vi "Profile Auton - Shooting Mode.vi"(8 "error in (no error)":errorcluster, 10 "Time (s)":dbl, 11 "Shooting Mode":T1(ring)) -> (0 "error out":errorcluster)   [LabVIEW 2017]
uses:
  <vilib>/Rock Robotics/WPI/Solenoid/WPI_SolenoidValue.ctl
  <vilib>/Rock Robotics/WPI/Utilities/WPI_GetSetVariantRefNum.vi
  <vilib>/Rock Robotics/WPI/Solenoid/WPI_SolenoidSetEnum.vi
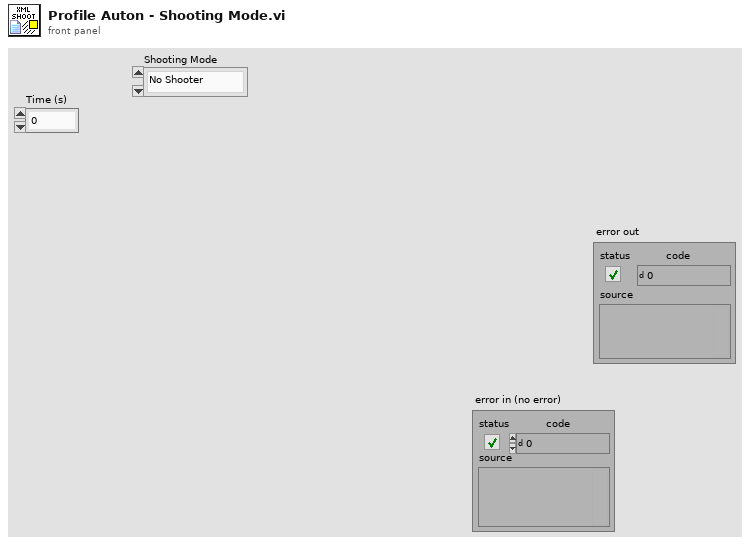
[diagram p1: front panel]
types:
  T1 = enum16{"No Shooter", "Switch Shooter", "Low Scale Shooter", "Mid Scale Shooter", "High Scale Shooter", "Reverse"}
  T2 = typedef "WPI_RobotDriveDevRef.ctl" = cluster{"DevStatus":errorcluster, "Motors[]":T3[], "Square Inputs":bool, "Max Output":dbl}
  T3 = typedef "WPI_MotorControlDeviceRef.ctl" = cluster{"DeviceStatus":errorcluster, "Type":T4, "PWM":cluster{"PWM Channel":T5, "DeadBand":T6}, "CAN":cluster{"Device Number":u8, "SetOutput VI Ref":variant, "GetOutput VI Ref":variant, "Enable VI Ref":variant, "Disable VI Ref":variant, "Data":variant}, "Invert":bool, "DIO PWM":cluster{"PWM \"Enable\" Channel":T5, "DIOChannel":T7, "PWM Rate":dbl}}
  T4 = typedef "WPI_MotorControlType.ctl" = enum16{"PWM", "CAN", "DIO PWM"}
  T5 = typedef "FPGA_DIOPWMChannel.ctl" = enum8{"PWM 0", "PWM 1", "PWM 2", "PWM 3", "PWM 4", "PWM 5", "PWM 6", "PWM 7", "PWM 8", "PWM 9", "PWM MXP 0", "PWM MXP 1", "PWM MXP 2", "PWM MXP 3", "PWM MXP 4", "PWM MXP 5", "PWM MXP 6", "PWM MXP 7", "PWM MXP 8", "PWM MXP 9", "Invalid"}
  T6 = typedef "WPI_PWMDeadband.ctl" = cluster{"Name":string, "maxPositivePwm":i32, "minPositivePwm":i32, "centerPwm":i32, "maxNegativePwm":i32, "minNegativePwm":i32, "angularRange":u16}
  T7 = typedef "FPGA_DIOChannel.ctl" = enum8{"DIO 0", "DIO 1", "DIO 2", "DIO 3", "DIO 4", "DIO 5", "DIO 6", "DIO 7", "DIO 8", "DIO 9", "DIO MXP 0", "DIO MXP 1", "DIO MXP 2", "DIO MXP 3", "DIO MXP 4", "DIO MXP 5", "DIO MXP 6", "DIO MXP 7", "DIO MXP 8", "DIO MXP 9", "DIO MXP 10", "DIO MXP 11", "DIO MXP 12", "DIO MXP 13", "DIO MXP 14", "DIO MXP 15", "SPI Port CS1", "SPI Port CS2", "SPI Port CS3", "SPI Port MISO", "SPI Port MOSI", "Invalid"}
  T8 = typedef "WPI_SolenoidDevRef.ctl" = cluster{"DevStatus":errorcluster, "Pneumatics Control Module":u8, "Forward Solenoid Channel":T9, "Reverse Solenoid Channel":T9}
  T9 = typedef "WPI_SolenoidChannel.ctl" = enum8{"Solenoid 0", "Solenoid 1", "Solenoid 2", "Solenoid 3", "Solenoid 4", "Solenoid 5", "Solenoid 6", "Solenoid 7", "Invalid"}
  T10 = typedef "WPI_SolenoidValue.ctl" = enum16{"Off", "On", "Forward", "Reverse"}
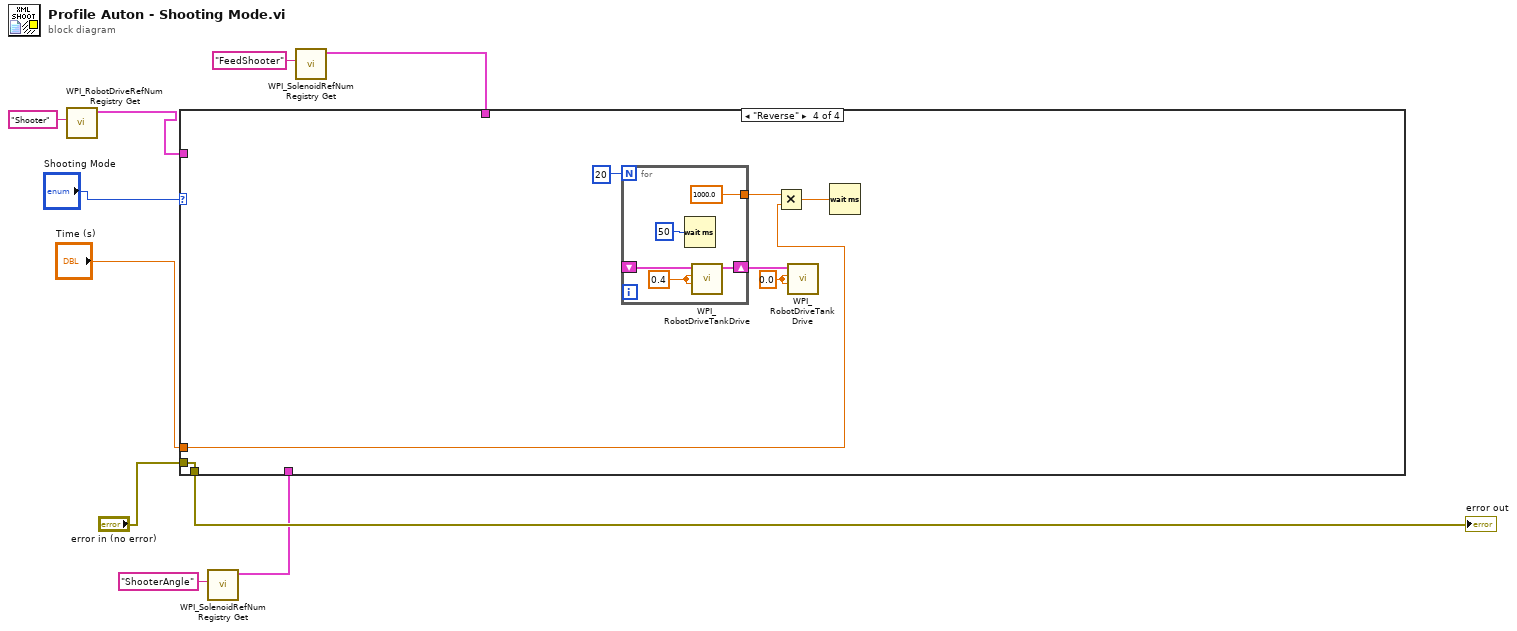
[diagram p0: block diagram]
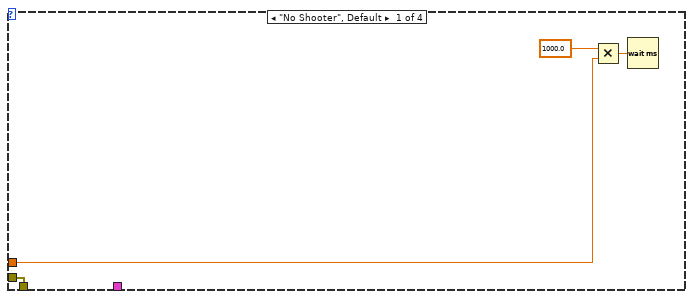
[diagram p2: hidden frame]
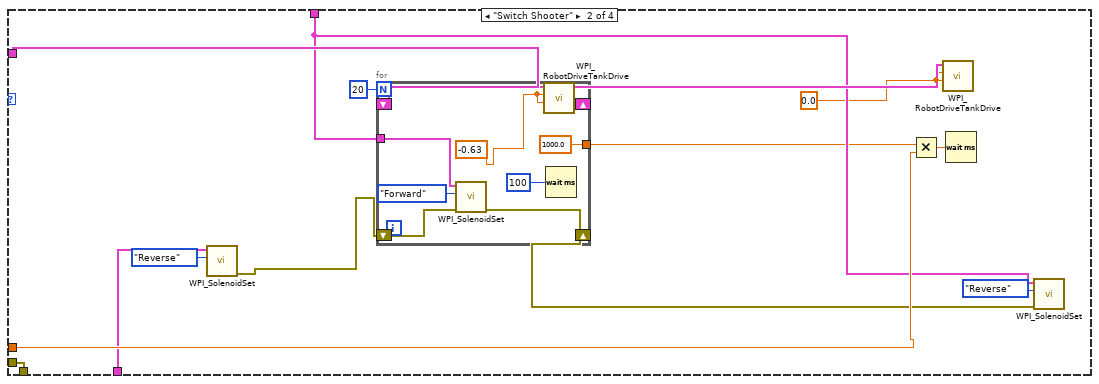
[diagram p3: hidden frame]
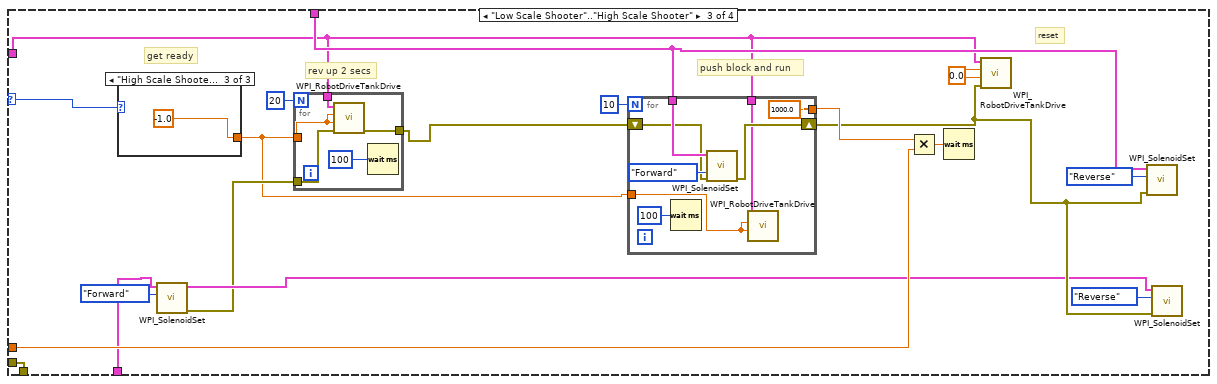
[diagram p4: hidden frame]
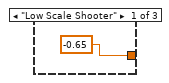
[diagram p5: hidden frame]
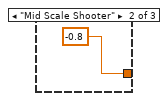
[diagram p6: hidden frame]
diagram:
  n1 = call <vilib>:"WPI_RobotDriveRefNum Registry Get.vi"("refnum name"="Shooter") -> ("RobotDriveDevRef"=w5:T2)  [unwired: 9 in, 1 out]
  n2 = call <vilib>:"WPI_SolenoidRefNum Registry Get.vi"("refnum name"="ShooterAngle") -> ("SolenoidDevRef"=w1:T8)  [unwired: 9 in, 1 out]
  n3 = call <vilib>:"WPI_SolenoidRefNum Registry Get.vi"("refnum name"="FeedShooter") -> ("SolenoidDevRef"=w2:T8)  [unwired: 9 in, 1 out]
  n4 = case shown="\"Reverse\"" "Shooting Mode" {
    selector: "Shooting Mode" -> [_ _ w54 _]
    tunnel: "Time (s)" -> [w12 w28 w56 w74]
    tunnel: "error in (no error)" -> [w11 w27 w55 w73]
    tunnel: [w11 w27 w55 w73] -> w8
    tunnel: w5 -> [_ w26 w39 _]
    tunnel: w2 -> [_ w22 w48 _]
    tunnel: w1 -> [_ w24 w47 _]
    frame "No Shooter", Default {
      n5 = Multiply(x=1000.0, y=w12) -> (x*y=w14:dbl)
      n6 = Wait (ms)(milliseconds to wait=w14) -> ()  [unwired: 1 out]
    }
    frame "Switch Shooter" {
      w19 = 0.0
      n7 = call-poly <vilib>:"WPI_SolenoidSet.vi"("Value"=WPI_SolenoidValue."Reverse", "SolenoidDevRef"=w24) -> ("error out"=w23:errorcluster)  [unwired: 8 in, 1 out]
      n8 = for {
        N: 20 -> [_]
        tunnel: w22 -> [w32]
        tunnel: [1000.0 ("x")] -> w17
        shift-right: [w34] -> w25
        shift-left: w26 -> [w35]
        shift-right: [w29] -> w16
        shift-left: w23 -> [w31]
        w36 = -0.63
        n9 = call-poly <vilib>:"WPI_SolenoidSet.vi"("error in (no error)"=w31, "Value"=WPI_SolenoidValue."Forward", "SolenoidDevRef"=w32) -> ("error out"=w29:errorcluster)  [unwired: 7 in, 1 out]
        n10 = call <vilib>:"WPI_RobotDriveTankDrive.vi"("Right axis value"=w36, "Left axis value"=w36, "RobotDriveDevRef"=w35) -> ("RobotDriveDevRef"=w34:T2)  [unwired: 6 in, 2 out]
        n11 = Wait (ms)(milliseconds to wait=u32 100) -> ()  [unwired: 1 out]
      }
      n12 = Multiply(x=w17, y=w28) -> (x*y=w20:dbl)
      n13 = call <vilib>:"WPI_RobotDriveTankDrive.vi"("Right axis value"=w19, "Left axis value"=w19, "RobotDriveDevRef"=w25) -> ()  [unwired: 6 in, 3 out]
      n14 = Wait (ms)(milliseconds to wait=w20) -> ()  [unwired: 1 out]
      n15 = call-poly <vilib>:"WPI_SolenoidSet.vi"("error in (no error)"=w16, "Value"=WPI_SolenoidValue."Reverse", "SolenoidDevRef"=w22) -> ()  [unwired: 7 in, 2 out]
    }
    frame "Low Scale Shooter".."High Scale Shooter" {
      w51 = 0.0
      # "push block and run"
      # "reset"
      # "rev up 2 secs"
      # "get ready"
      n16 = case shown="\"High Scale Shooter\", Default" w54 {
        tunnel: [-0.65 -0.8 -1.0] -> w40
        frame "Low Scale Shooter" {
        }
        frame "Mid Scale Shooter" {
        }
        frame "High Scale Shooter", Default {
        }
      }
      n17 = call-poly <vilib>:"WPI_SolenoidSet.vi"("Value"=WPI_SolenoidValue."Forward", "SolenoidDevRef"=w47) -> ("error out"=w43:errorcluster, "SolenoidDevRef"=w44:T8)  [unwired: 8 in]
      n18 = for {
        N: 20 -> [_]
        tunnel: w39 -> [w68]
        tunnel: w40 -> [w67]
        tunnel: w43 -> [w66]
        tunnel: [w65] -> w42
        n19 = call <vilib>:"WPI_RobotDriveTankDrive.vi"("error in (no error)"=w66, "Right axis value"=w67, "Left axis value"=w67, "RobotDriveDevRef"=w68) -> ("error out"=w65:errorcluster)  [unwired: 5 in, 2 out]
        n20 = Wait (ms)(milliseconds to wait=u32 100) -> ()  [unwired: 1 out]
      }
      n21 = for {
        N: 10 -> [_]
        tunnel: w48 -> [w64]
        tunnel: [1000.0 ("x")] -> w46
        shift-right: [w61] -> w45
        shift-left: w42 -> [w62]
        tunnel: w40 -> [w58]
        tunnel: w39 -> [w57]
        n22 = Wait (ms)(milliseconds to wait=u32 100) -> ()  [unwired: 1 out]
        n23 = call-poly <vilib>:"WPI_SolenoidSet.vi"("error in (no error)"=w62, "Value"=WPI_SolenoidValue."Forward", "SolenoidDevRef"=w64) -> ("error out"=w61:errorcluster)  [unwired: 7 in, 1 out]
        n24 = call <vilib>:"WPI_RobotDriveTankDrive.vi"("Right axis value"=w58, "Left axis value"=w58, "RobotDriveDevRef"=w57) -> ()  [unwired: 6 in, 3 out]
      }
      n25 = Multiply(x=w46, y=w56) -> (x*y=w52:dbl)
      n26 = Wait (ms)(milliseconds to wait=w52) -> ()  [unwired: 1 out]
      n27 = call <vilib>:"WPI_RobotDriveTankDrive.vi"("error in (no error)"=w45, "Right axis value"=w51, "Left axis value"=w51, "RobotDriveDevRef"=w39) -> ()  [unwired: 5 in, 3 out]
      n28 = call-poly <vilib>:"WPI_SolenoidSet.vi"("error in (no error)"=w45, "Value"=WPI_SolenoidValue."Reverse", "SolenoidDevRef"=w48) -> ()  [unwired: 7 in, 2 out]
      n29 = call-poly <vilib>:"WPI_SolenoidSet.vi"("error in (no error)"=w45, "Value"=WPI_SolenoidValue."Reverse", "SolenoidDevRef"=w44) -> ()  [unwired: 7 in, 2 out]
    }
    frame "Reverse" {
      w77 = 0.0
      n30 = for {
        N: 20 -> [_]
        tunnel: [1000.0 ("x")] -> w76
        shift-right: [w81] -> w79
        shift-left: _ -> [w82]
        w83 = 0.4
        n31 = Wait (ms)(milliseconds to wait=u32 50) -> ()  [unwired: 1 out]
        n32 = call <vilib>:"WPI_RobotDriveTankDrive.vi"("Right axis value"=w83, "Left axis value"=w83, "RobotDriveDevRef"=w82) -> ("RobotDriveDevRef"=w81:T2)  [unwired: 6 in, 2 out]
      }
      n33 = Multiply(x=w76, y=w74) -> (x*y=w78:dbl)
      n34 = call <vilib>:"WPI_RobotDriveTankDrive.vi"("Right axis value"=w77, "Left axis value"=w77, "RobotDriveDevRef"=w79) -> ()  [unwired: 6 in, 3 out]
      n35 = Wait (ms)(milliseconds to wait=w78) -> ()  [unwired: 1 out]
    }
  }
  "error out" <- w8
